vi "Pull out Scale Info_NET.vi"(8 "error in":errorcluster, 11 "reference in":T2) -> (0 "error out":errorcluster, 3 "Scale Info":T1)   [LabVIEW 2019, in "J1939 Workspace Object.lvlib"]
uses:
  J1939 Workspace Object.lvlib
  <vilib>/NI VeriStand/UI Controls/Single Node Browser/Node Ref.ctl
  NationalInstruments.VeriStand.SystemStorage
  Shared/Types/SPN Properties.ctl
  Shared/SubVIs/Constants.vi
  Shared/J1939 Addon Shared.lvlib
  <vilib>/NI VeriStand/UI Controls/Single Node Browser/NI_VS UI Single Node Browser.lvlib
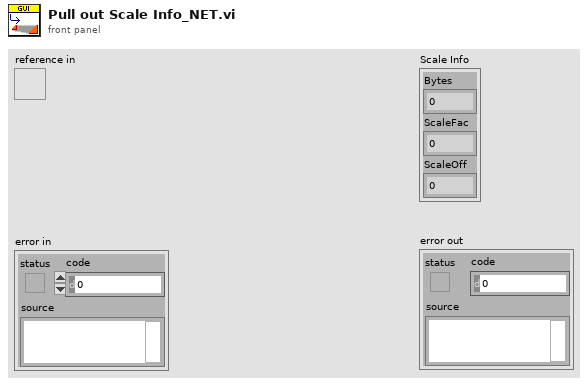
[diagram p1: front panel]
types:
  T1 = typedef "J1939 Addon Shared.lvlib/SPN Properties.ctl" = cluster{"Bytes":u32, "ScaleFac":dbl, "ScaleOff":dbl}
  T2 = typedef "NI_VS UI Single Node Browser.lvlib/Node Ref.ctl" = refnum<k24>
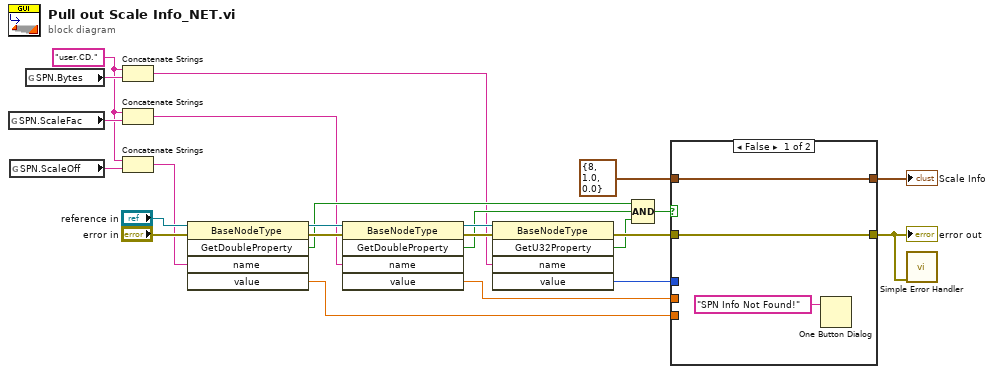
[diagram p0: block diagram]
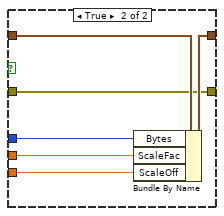
[diagram p2: hidden frame]
diagram:
  w1 = "user.CD." ("string")
  n1 = global read "Constants.vi" "SPN.ScaleFac"() -> (w12:string)
  n2 = global read "Constants.vi" "SPN.ScaleOff"() -> (w11:string)
  n3 = global read "Constants.vi" "SPN.Bytes"() -> (w15:string)
  n4 = Concatenate Strings(w1, w15) -> (w4:string)
  n5 = Concatenate Strings(w1, w12) -> (w3:string)
  n6 = Concatenate Strings(w1, w11) -> (w2:string)
  n7 = invoke class="BaseNodeType" method="GetDoubleProperty"(reference="reference in", error in="error in", "name"=w2) -> (reference out=w18:T2, error out=w19:errorcluster, "GetDoubleProperty"=w7:bool, "value"=w13:dbl)  [unwired: 2 in, 1 out]
  n8 = invoke class="BaseNodeType" method="GetDoubleProperty"(reference=w18, error in=w19, "name"=w3) -> (reference out=w16:T2, error out=w17:errorcluster, "GetDoubleProperty"=w8:bool, "value"=w14:dbl)  [unwired: 2 in, 1 out]
  n9 = invoke class="BaseNodeType" method="GetU32Property"(reference=w16, error in=w17, "name"=w4) -> (error out=w21:errorcluster, "GetU32Property"=w6:bool, "value"=w20:u32)  [unwired: 2 in, 2 out]
  n10 = Compound Arithmetic op=AND(w7, w8, w6) -> (w5:bool)
  n11 = case shown="False" w5 {
    tunnel: [w27 w31] -> w24
    tunnel: T1 {"Bytes"=8, "ScaleFac"=1.0, "ScaleOff"=0.0} ("cluster") -> [w26 w33]
    tunnel: [w26 w32] -> w22
    tunnel: w21 -> [w27 w31]
    tunnel: w20 -> [_ w30]
    tunnel: w14 -> [_ w29]
    tunnel: w13 -> [_ w28]
    frame False {
      n12 = One Button Dialog(message="SPN Info Not Found!") -> ()  [unwired: 1 in, 1 out]
    }
    frame True {
      n13 = Bundle By Name(cluster=w33, "Bytes"=w30, "ScaleFac"=w29, "ScaleOff"=w28) -> (w32:T1)
    }
  }
  "error out" <- w24
  "Scale Info" <- w22
  n14 = call <vilib>:"Simple Error Handler.vi"("error in (no error)"=w24) -> ()  [unwired: 4 in, 5 out]
